vi "ND Engine.vi"() -> ()   [LabVIEW 2013]
uses:
  Classes/GanntChart.lvclass
panel:
  out "Start Times":u16[][](array[numeric])
  out "Schedule Order":u16[](array[numeric])
  out "Schedule":u16[](array[numeric])
  out "Machine Completion Time":u16[](array[numeric])
  out "Job Completion Times":u16[](array[numeric])
  out "Completion Times":u16[][](array[numeric])
  in  "Number of  Jobs":i32=4
  in  "Number of Machines":i32=4
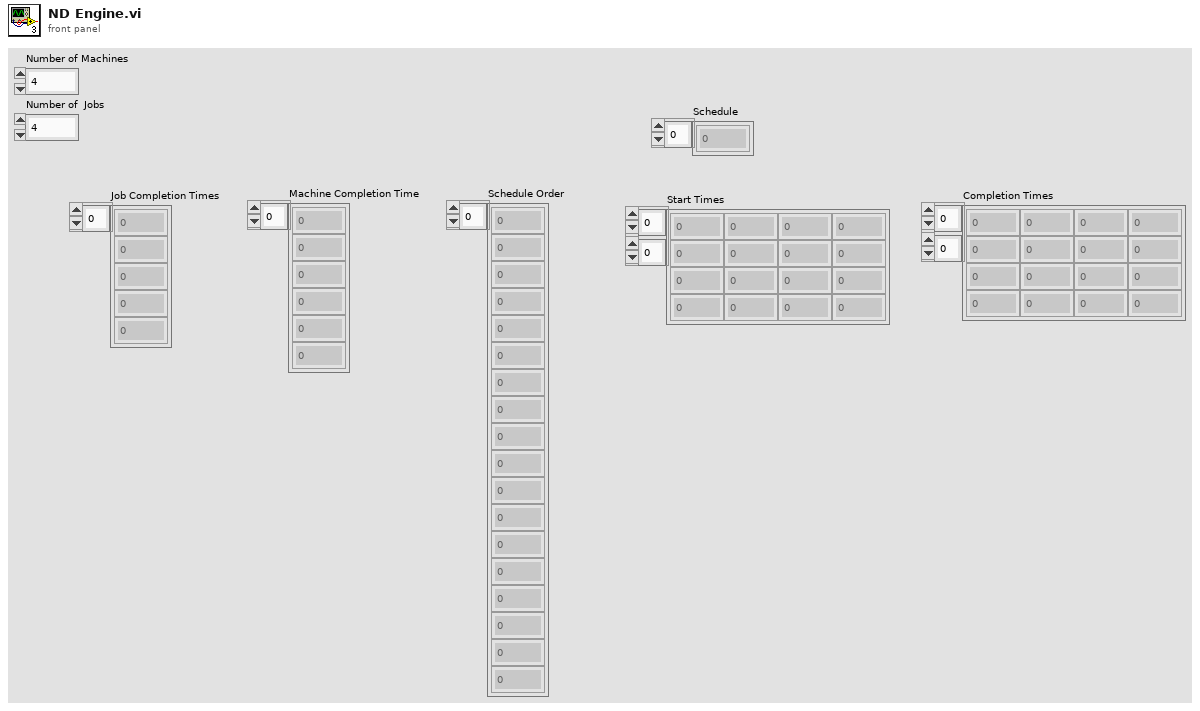
[diagram p1: front panel]
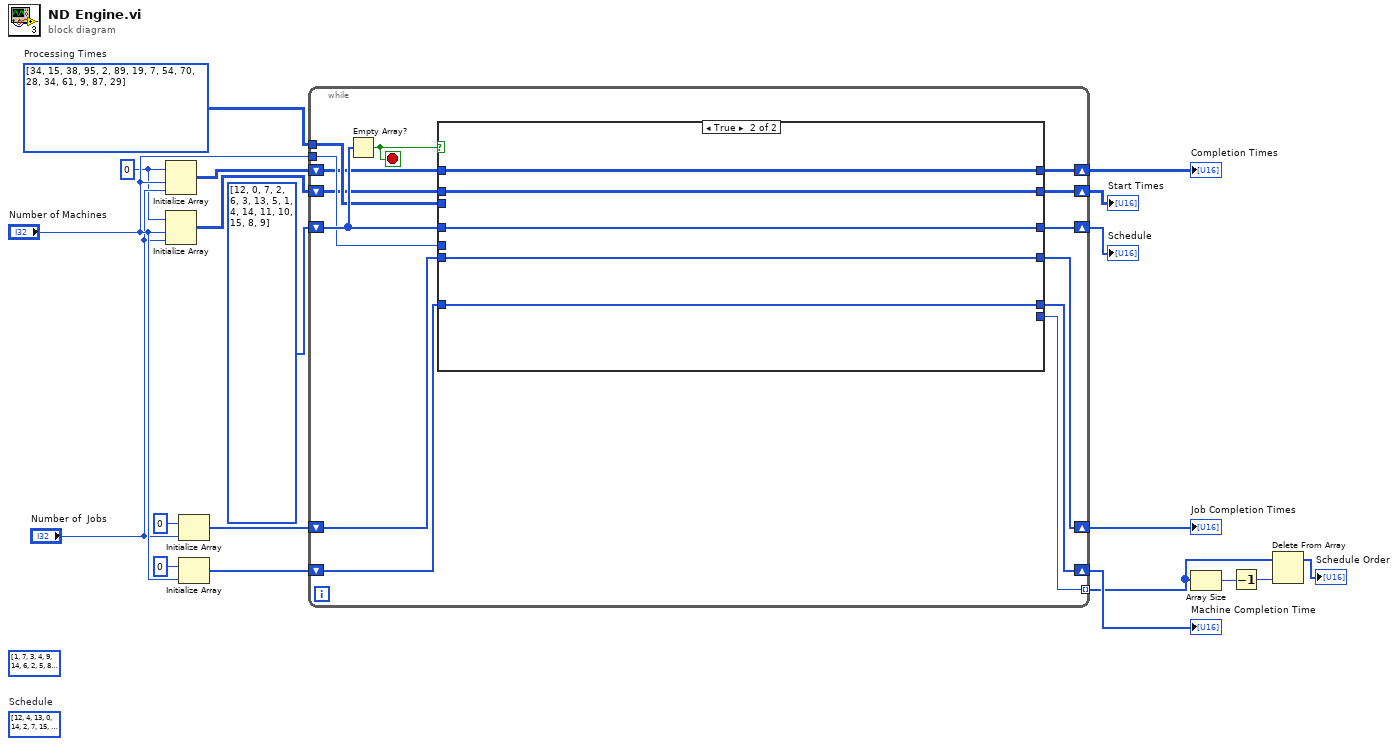
[diagram p0: block diagram]
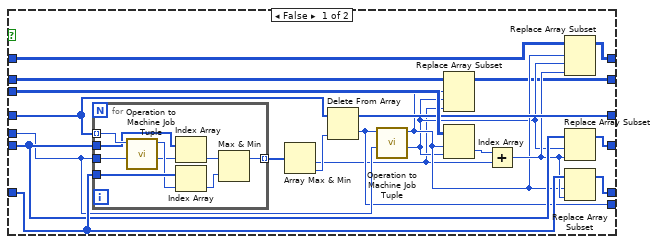
[diagram p2: hidden frame]
diagram:
  (unwired) u16[] [1, 7, 3, 4, 9, 14, 6, 2, 5, 8, 13, 11, 0, 12, 10, 15] ("Schedule")
  w3 = u16 0 ("element")
  w16 = u16[][] [[34, 15, 38, 95], [2, 89, 19, 7], [54, 70, 28, 34], [61, 9, 87, 29]]  # Processing Times
  (unwired) u16[] [12, 4, 13, 0, 14, 2, 7, 15, 9, 1, 6, 3, 11, 10, 5, 8]  # Schedule
  n1 = Initialize Array(w3, "Number of Machines", "Number of  Jobs") -> (w15:u16[][])
  n2 = Initialize Array(w3, "Number of Machines", "Number of  Jobs") -> (w2:u16[][])
  n3 = Initialize Array(u16 0 ("element"), "Number of  Jobs") -> (w18:u16[])
  n4 = Initialize Array(u16 0 ("element"), "Number of Machines") -> (w17:u16[])
  n5 = while {
    shift-right: [w26] -> w11
    shift-left: u16[] [12, 0, 7, 2, 6, 3, 13, 5, 1, 4, 14, 11, 10, 15, 8, 9] -> [w33]
    tunnel: "Number of Machines" -> [w32]
    shift-right: [w29] -> w13
    shift-left: w18 -> [w31]
    shift-right: [w28] -> w12
    shift-left: w17 -> [w30]
    shift-right: [w24] -> w14
    shift-left: w15 -> [w25]
    tunnel: w16 -> [w27]
    tunnel: [w23] -> w9 mode=indexing
    shift-right: [w21] -> w1
    shift-left: w2 -> [w22]
    stop <- w34 stop-if-true
    n6 = Empty Array?(array=w33) -> (empty?=w34:bool)
    n7 = case shown="True" w34 {
      tunnel: w33 -> [w46 w66]
      tunnel: w32 -> [w41 _]
      tunnel: w31 -> [w52 w68]
      tunnel: w30 -> [w53 w67]
      tunnel: [w51 w68] -> w29
      tunnel: [w50 w67] -> w28
      tunnel: w27 -> [w54 _]
      tunnel: [w45 w66] -> w26
      tunnel: w25 -> [w49 w65]
      tunnel: [w48 w65] -> w24
      tunnel: [w40 _] -> w23
      tunnel: w22 -> [w39 w64]
      tunnel: [w35 w64] -> w21
      frame False {
        n8 = for {
          tunnel: w46 -> [w63] mode=indexing
          tunnel: w41 -> [w62]
          tunnel: w52 -> [w59]
          tunnel: w53 -> [w61]
          tunnel: [w55] -> w47 mode=indexing
          n9 = call "Operation to Machine Job Tuple.vi"("Number of Machines"=w62, "Operation Number"=w63) -> ("Job No"=w58:i32, "Machine No"=w60:i32)  [unwired: 8 in]
          n10 = Index Array(array=w59, index=w58) -> (element=w57:u16)
          n11 = Index Array(array=w61, index=w60) -> (element=w56:u16)
          n12 = Max & Min(x=w57, y=w56) -> (max(x,y)=w55:u16)  [unwired: 1 out]
        }
        n13 = Array Max & Min(array=w47) -> (min value=w36:u16, min index (indices)=w42:i32)  [unwired: 2 out]
        n14 = Delete From Array(array=w46, index=w42) -> (deleted portion=w40:u16, array with subset deleted=w45:u16[])  [unwired: 1 in]
        n15 = call "Operation to Machine Job Tuple.vi"("Number of Machines"=w41, "Operation Number"=w40) -> ("Job No"=w37:i32, "Machine No"=w38:i32)  [unwired: 8 in]
        n16 = Replace Array Subset(array=w39, new element=w36, index (row)=w38, index (col)=w37) -> (w35:u16[][])
        n17 = Index Array(array=w54, index (row)=w38, index (col)=w37) -> (element=w44:u16)
        n18 = Add(x=w44, y=w36) -> (x+y=w43:u16)
        n19 = Replace Array Subset(array=w49, new element=w43, index (row)=w38, index (col)=w37) -> (w48:u16[][])
        n20 = Replace Array Subset(array=w52, new element=w43, index=w37) -> (w51:u16[])
        n21 = Replace Array Subset(array=w53, new element=w43, index=w38) -> (w50:u16[])
      }
      frame True {
      }
    }
  }
  "Completion Times" <- w14
  "Job Completion Times" <- w13
  "Machine Completion Time" <- w12
  "Schedule" <- w11
  "Start Times" <- w1
  n22 = Array Size(array=w9) -> (size(s)=w8:i32)
  n23 = Decrement(x=w8) -> (x-1=w7:i32)
  n24 = Delete From Array(array=w9, index=w7) -> (array with subset deleted=→"Schedule Order":u16[])  [unwired: 1 in, 1 out]
